vi "Core Read DAQ FIFO.vi"(8 "error in (no error)":errorcluster, 9 "Timeout (ms)":i32, 11 "CIFFIFO in":refnum<class "CIF_CIPC_Fifo_DAQ.lvclass">) -> (0 "error out":errorcluster, 1 "timed out?":bool, 3 "CIFFIFO out":refnum<class "CIF_CIPC_Fifo_DAQ.lvclass">)   [LabVIEW 2021, in "CIF_CIPC_Fifo_DAQ.lvclass"]
uses:
  CIF_CIPC_Fifo_DAQ.lvclass
  D:/dev/Packages/CIF_Channels_Core/src/CIFChannels/CIFChannels.lvclass
  D:/dev/Packages/CIF_Channels_Core/src/CIPC_Channels/CIF_CIPC_Chan/CIF_CIPC_Chn.lvclass
  ChannelCommon/typedef/Channel State.ctl
  ChannelCommon/typedef/Direction.ctl
  CIFChannels/CIFChannels.lvclass/CIFChannels.ctl
  <vilib>/CIF Foundation/CIF CIPC/TypeDefs/Data Element Details.ctl
  <vilib>/CIF Foundation/CIF CIPC/TypeDefs/Read Configuration.ctl
  <vilib>/CIF Foundation/CIF CIPC/TypeDefs/Read Position.ctl
  CIF_CIPC_Chan/CIF_CIPC_Chn.lvclass/CIF_CIPC_Chn.ctl
  CIF_CIPC_Fifo_DAQ.lvclass/CIF_CIPC_Fifo_DAQ.ctl
  <vilib>/CIF Foundation/CIF Utilities/Statistics/I64/Stats_I64_CIF_U.lvclass/Stats_I64_CIF_U.ctl
  e703c505-0034-46a9-8989-21c0de27793f.vi
  768488f4-e6df-4560-a449-a64b33b49031.vi
  CIFChannels/Accessors/Read Channel State.vi
  CIFChannels/Accessors/Read Direction.vi
  <vilib>/CIF Foundation/CIF Utilities/DataTypes/Flatten Unflatten/Unflatten U64.vi
  <vilib>/CIF Foundation/CIF Utilities/DataTypes/Flatten Unflatten/Unflatten I64.vi
  ChannelCommon/Utilities/Add Error.vi
  Read Wrapper for BP Meta.vi
  Read Wrapper for BP Measurements.vi
  CIF_CIPC_Chan/Accessors/Read CIPC Channel.vi
  Read Wrapper for BP U8.vi/b5615cf0-cd7f-4476-b9a9-d6ef7628cc3b.vi
  CIF_CIPC_Chan/Accessors/Read Buffer Configuration.vi
  Read Wrapper for BP U8.vi/6248fc70-cc83-4025-b778-a3221b95feac.vi
  CIFChannels/Accessors/Read FIFO Backpressure.vi
  <vilib>/CIF Foundation/CIF Utilities/Statistics/I64/X1 minus X0.vi
  <vilib>/CIF Foundation/CIF Utilities/Time/System Time/Get System Time.vi
  Read Wrapper for BP Meta.vi/b5615cf0-cd7f-4476-b9a9-d6ef7628cc3b.vi
  Read Wrapper for BP Meta.vi/6248fc70-cc83-4025-b778-a3221b95feac.vi
  Read Wrapper for BP Measurements.vi/b5615cf0-cd7f-4476-b9a9-d6ef7628cc3b.vi
  Read Wrapper for BP Measurements.vi/6248fc70-cc83-4025-b778-a3221b95feac.vi
  <vilib>/CIF Foundation/CIF CIPC/SubVIs/Wait For N Elements Available.vi
  <vilib>/CIF Foundation/CIF CIPC/SubVIs/Get Element Read Position.vi
  <vilib>/CIF Foundation/CIF CIPC/SubVIs/Check Error.vi
  <vilib>/CIF Foundation/CIF CIPC/SubVIs/Get dll Path.vi
  <vilib>/CIF Foundation/CIF CIPC/SubVIs/Set Element Read Position.vi
  Read Wrapper for BP U8.vi/6248fc70-cc83-4025-b778-a3221b95feac.vi/331f6ecb-7ec4-4931-b93d-4fbd8d66a851.vi
  Read Wrapper for BP U8.vi/6248fc70-cc83-4025-b778-a3221b95feac.vi/5ce0d4cf-f921-42ba-b14c-c90f7f7611e4.vi
  <vilib>/CIF Foundation/CIF Utilities/Statistics/I64/X1 minus X0.vi/dfabcf33-0dbc-4041-80a5-3dc0c86d2989.vi
  <vilib>/CIF Foundation/CIF Utilities/Time/System Time/LabVIEW Time to TAI Time.vi
  Read Wrapper for BP Meta.vi/6248fc70-cc83-4025-b778-a3221b95feac.vi/331f6ecb-7ec4-4931-b93d-4fbd8d66a851.vi
  Read Wrapper for BP Meta.vi/6248fc70-cc83-4025-b778-a3221b95feac.vi/5ce0d4cf-f921-42ba-b14c-c90f7f7611e4.vi
  Read Wrapper for BP Measurements.vi/6248fc70-cc83-4025-b778-a3221b95feac.vi/331f6ecb-7ec4-4931-b93d-4fbd8d66a851.vi
  Read Wrapper for BP Measurements.vi/6248fc70-cc83-4025-b778-a3221b95feac.vi/5ce0d4cf-f921-42ba-b14c-c90f7f7611e4.vi
  <vilib>/CIF Foundation/CIF CIPC/SubVIs/Notify Of New Write.vi
  <vilib>/CIF Foundation/CIF CIPC/SubVIs/Get Element Write Position.vi
  <vilib>/CIF Foundation/CIF Utilities/Statistics/I64/X1 minus X0.vi/dfabcf33-0dbc-4041-80a5-3dc0c86d2989.vi/9eb60a9a-770f-4d2d-8b3f-8465c267ecc9.vi
  <vilib>/CIF Foundation/CIF CIPC/SubVIs/Check Error Core.vi
  <vilib>/CIF Foundation/CIF CIPC/SubVIs/Get Element Info Variant.vi
  ChannelCommon/Utilities/Add Error Core.vi
  ChannelCommon/ChannelCommon.lvlib
  CIFChannels/CIFChannels.lvclass
  <vilib>/CIF Foundation/CIF CIPC/CIF_NI_CIPC.lvlib
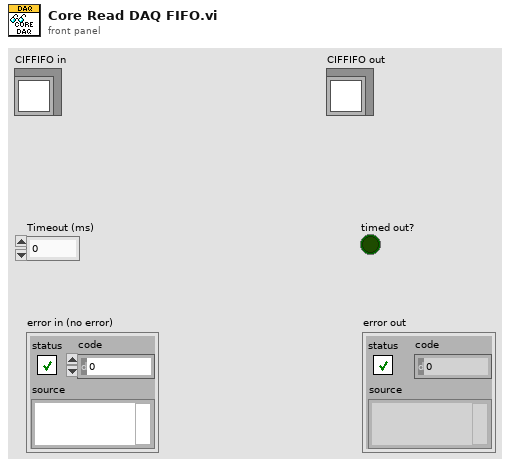
[diagram p1: front panel]
types:
  T1 = typedef "ChannelCommon.lvlib/Channel State.ctl" = enum8{"Creating", "Disconnected", "Connecting", "Connected", "Destroyed"}
  T2 = typedef "ChannelCommon.lvlib/Direction.ctl" = enum8{"Publisher", "Subscriber"}
  T3 = typedef "CIF_NI_CIPC.lvlib/Data Element Details.ctl" = cluster{"Bytes to Read":u32, "Element Offset":u32}
  T4 = typedef "CIF_NI_CIPC.lvlib/Read Configuration.ctl" = cluster{"Read Position":T5, "Element Offset":i32, "Prepend Array Size":bool, "Get Read Position":bool}
  T5 = typedef "CIF_NI_CIPC.lvlib/Read Position.ctl" = enum8{"Next", "Newest", "Oldest", "Next Available", "Absolute"}
  T6 = typedef "ChannelCommon.lvlib/FIFO Header.ctl" = cluster{"Length":u64, "T0":i64, "T_Out":i64, "T_Tx":i64, "Ctr":u64, "ClockID":u8}
  T7 = typedef "ChannelCommon.lvlib/Datatype Waveform.ctl" = cluster{"Measurement":dbl[], "dT":dbl, "Timestamp":i64}
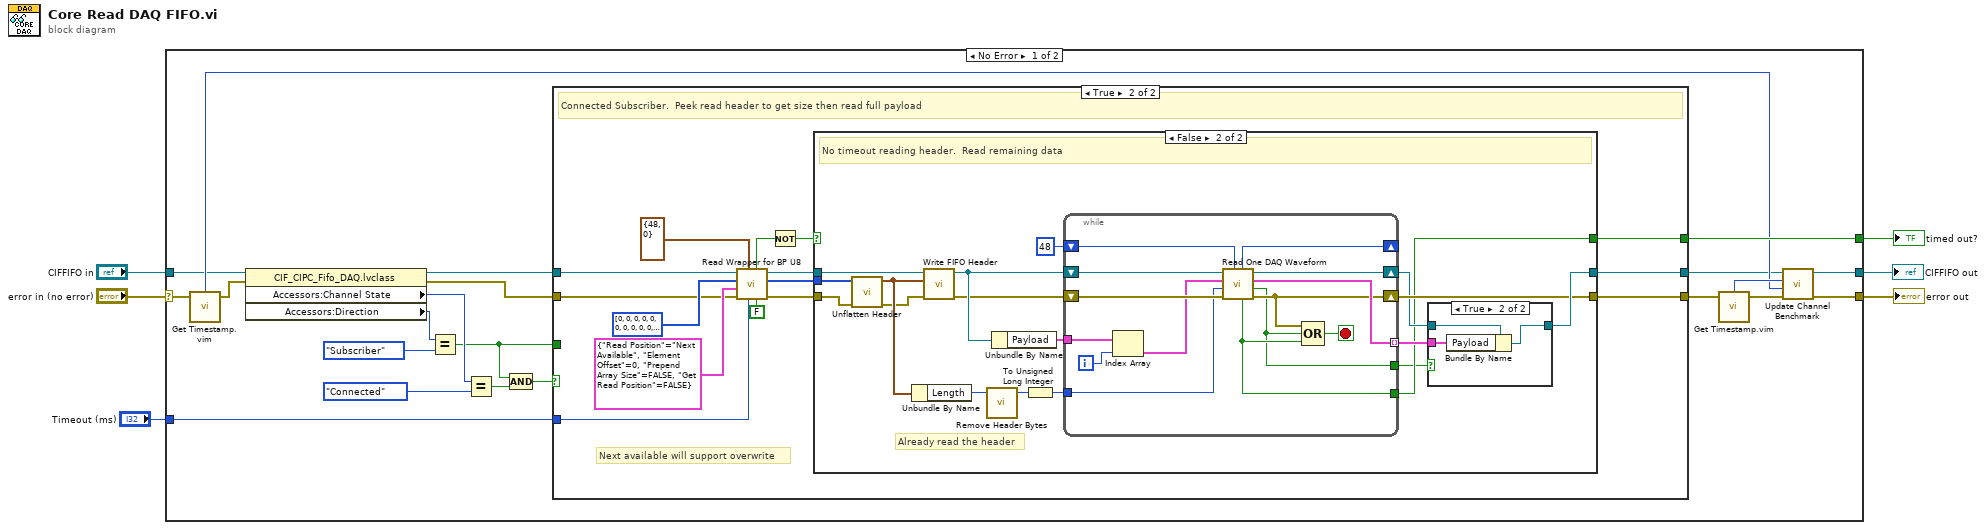
[diagram p0: block diagram]
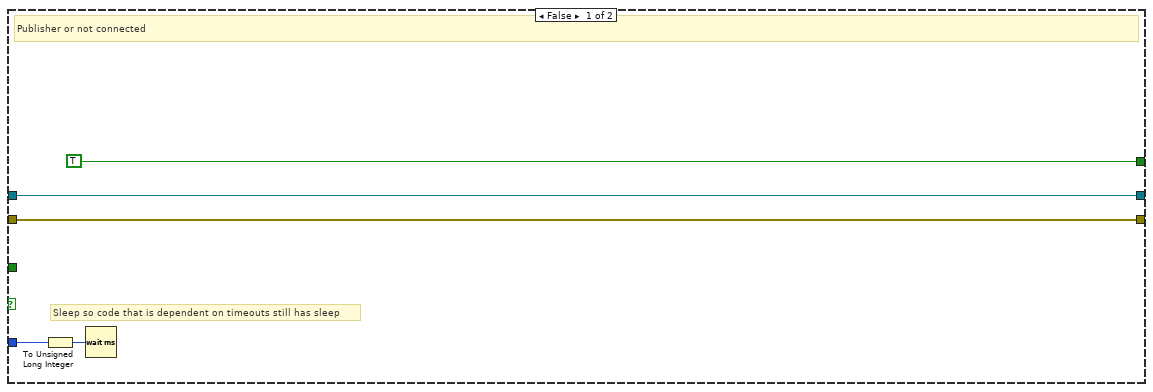
[diagram p2: hidden frame]
diagram:
  n1 = case shown="No Error" "error in (no error)" {
    selector: "error in (no error)" -> [w9 w88]
    tunnel: [w15 w88] -> w1
    tunnel: [w16 w87] -> w2
    tunnel: "CIFFIFO in" -> [w8 w87]
    tunnel: [w27 _] -> w3
    tunnel: "Timeout (ms)" -> [w17 _]
    frame No Error {
      n2 = call "Get Timestamp.vim"("Anything in"=w9) -> ("Time (ns)"=w13:i64, "Anything out"=w7:errorcluster)  [unwired: 2 in]
      n3 = property class="CIF_CIPC_Fifo_DAQ.lvclass"(reference=w8, error in=w7) -> (reference out=w26:refnum<class "CIF_CIPC_Fifo_DAQ.lvclass">, error out=w25:errorcluster, "Accessors:Channel State"=w22:T1, "Accessors:Direction"=w24:T2)
      n4 = Equal?(x=w24, y=Direction."Subscriber") -> (x = y?=w18:bool)
      n5 = Equal?(x=w22, y=Channel_State."Connected") -> (x = y?=w20:bool)
      n6 = Compound Arithmetic op=AND(w18, w20) -> (w19:bool)
      n7 = case shown="True" w19 {
        tunnel: [TRUE ("timeout out") w34] -> w27
        tunnel: w25 -> [w31 w38]
        tunnel: w26 -> [w32 w33]
        tunnel: w18 -> [_ _]
        tunnel: [w32 w47] -> w11
        tunnel: [w31 w46] -> w10
        tunnel: w17 -> [w29 w41]
        frame False {
          # "Sleep so code that is dependent on timeouts still has sleep"
          # "Publisher or not connected"
          n8 = To Unsigned Long Integer(number=w29) -> (unsigned 32bit integer=w28:u32)
          n9 = Wait (ms)(milliseconds to wait=w28) -> ()  [unwired: 1 out]
        }
        frame True {
          # "Next available will support overwrite"
          # "Connected Subscriber.  Peek read header to get size then read full payload"
          n10 = call "Read Wrapper for BP U8.vi"("Last Read"=FALSE, "Timeout (ms)"=w41, "Data Element"=T3 {"Bytes to Read"=48, "Element Offset"=0}, "error in (no error)"=w38, "Read Configuration"=T4 {"Read Position"=enum."Next Available", "Element Offset"=0, "Prepend Array Size"=FALSE, "Get Read Position"=FALSE}, "Data in"=u8[] [0, 0, 0, 0, 0, 0, 0, 0, 0, 0, 0, 0, 0, 0, 0, 0, 0, 0, 0, 0, 0, 0, 0, 0, 0, 0, 0, 0, 0, 0, 0, 0, 0, 0, 0, 0, 0, 0, 0, 0, 0, 0, 0, 0, 0, 0, 0, 0] ("U8 Array in"), "CIF_CIPC_Fifo_U8 in"=w33) -> ("error out"=w40:errorcluster, "Data out"=w39:u8[], "CIF_CIPC_Fifo_U8 out"=w45:refnum<class "CIF_CIPC_Fifo_DAQ.lvclass">, "Success"=w36:bool)  [unwired: 1 out]
          n11 = Not(x=w36) -> (.not. x?=w35:bool)
          n12 = case shown="False" w35 {
            selector: w35 -> [w48 _]
            tunnel: w45 -> [w50 w66]
            tunnel: w40 -> [w49 w68]
            tunnel: w39 -> [_ w67]
            tunnel: [w49 w56] -> w46
            tunnel: [w50 w63] -> w47
            tunnel: [w48 w54] -> w34
            frame True {
              # "Timeout reading header"
            }
            frame False {
              # "Already read the header"
              # "No timeout reading header.  Read remaining data"
              n13 = call "Unflatten Header.vi"("error in (no error)"=w68, "Flattened Data in"=w67) -> ("error out"=w64:errorcluster, "Header out"=w65:T6)  [unwired: 7 in, 1 out]
              n14 = Unbundle By Name(w65) -> ("Length"=w62:u64)
              n15 = call "Write FIFO Header.vi"("error in (no error)"=w64, "Header"=w65, "CIFChannels in"=w66) -> ("error out"=w58:errorcluster, "CIFChannels out"=w60:refnum<class "CIF_CIPC_Fifo_DAQ.lvclass">)  [unwired: 7 in]
              n16 = call "Remove Header Bytes.vi"("Bytes/Msg with header"=w62) -> ("Bytes/Msg without header"=w61:u64)  [unwired: 3 in]
              n17 = Unbundle By Name(w60) -> ("Payload"=w59:T7[])
              n18 = To Unsigned Long Integer(number=w61) -> (unsigned 32bit integer=w52:u32)
              n19 = while {
                tunnel: w59 -> [w75]
                shift-right: [w84] -> w55
                shift-left: w60 -> [w86]
                shift-right: [w82] -> w56
                shift-left: w58 -> [w85]
                tunnel: [w83] -> w57 mode=indexing
                tunnel: [w80] -> w54
                tunnel: [w79] -> w53
                tunnel: w52 -> [w78]
                shift-right: [w77] -> _
                shift-left: u32 48 ("Offset out") -> [w76]
                i -> [w74]
                stop <- w81 stop-if-true
                n20 = Index Array(array=w75, index=w74) -> (element=w73:T7)
                n21 = call "Read One DAQ Waveform.vi"("Offset in"=w76, "error in (no error)"=w85, "Total Length"=w78, "Waveform Datatype in"=w73, "CIF_CIPC_Fifo_U8 in"=w86) -> ("error out"=w82:errorcluster, "Done"=w79:bool, "Waveform Datatype out"=w83:T7, "CIF_CIPC_Fifo_U8 out"=w84:refnum<class "CIF_CIPC_Fifo_DAQ.lvclass">, "Timeout"=w80:bool, "Offset out"=w77:u32)  [unwired: 1 in]
                n22 = Compound Arithmetic op=OR(w82, w79, w80) -> (w81:bool)
              }
              n23 = case shown="True" w53 {
                tunnel: [w69 w72] -> w63
                tunnel: w57 -> [_ w71]
                tunnel: w55 -> [w69 w70]
                frame False {
                }
                frame True {
                  n24 = Bundle By Name(cluster=w70, "Payload"=w71) -> (w72:refnum<class "CIF_CIPC_Fifo_DAQ.lvclass">)
                }
              }
            }
          }
        }
      }
      n25 = call "Get Timestamp.vim"("Anything in"=w10) -> ("Time (ns)"=w14:i64, "Anything out"=w12:errorcluster)  [unwired: 2 in]
      n26 = call "Update Channel Benchmark.vi"("error in (no error)"=w12, "X0"=w13, "X1"=w14, "CIFChannels in"=w11) -> ("error out"=w15:errorcluster, "CIFChannels out"=w16:refnum<class "CIF_CIPC_Fifo_DAQ.lvclass">)  [unwired: 6 in]
    }
    frame Error {
    }
  }
  "error out" <- w1
  "timed out?" <- w3
  "CIFFIFO out" <- w2
